vi "BuildExe.vi"(8 "Error In":errorcluster, 9 "Version number":T1, 10 "Build specification name":string, 11 "Path":path) -> (0 "Error Out":errorcluster)   [LabVIEW 2019]
uses:
  <vilib>/AppBuilder/AB_API/common/AB_API Version Number.ctl
  <vilib>/AppBuilder/AB_API/common/AB_API Build Object Selector.ctl
  <vilib>/AppBuilder/AB_API/Build/NI_AB_API_Build.lvclass
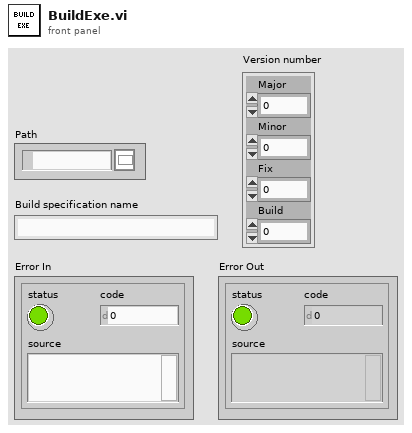
[diagram p1: front panel]
types:
  T1 = typedef "AB_API Version Number.ctl" = cluster{"Major":u16, "Minor":u16, "Fix":u16, "Build":u16}
  T2 = typedef "AB_API Build Object Selector.ctl" = enum16{"Source Distribution", "Deployable Source Distribution", "DLL", "EXE", "Packed Library", "Deployable Packed Library", "RT EXE", ".NET Interop Assembly"}
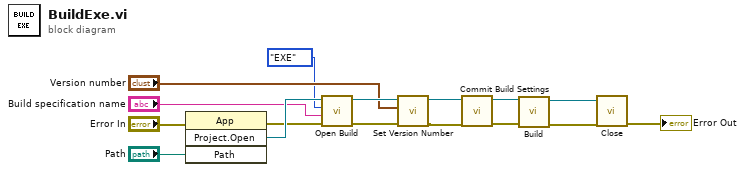
[diagram p0: block diagram]
diagram:
  n1 = invoke class="App" method="Project.Open"(error in="Error In", "Path"="Path") -> (error out=w13:errorcluster, "Project:Open"=w15:refnum<vi>)  [unwired: 2 in, 2 out]
  n2 = call <vilib>:"Open Build.vi"("error in (no error)"=w13, "Build specification name"="Build specification name", "Build object selector"=AB_API_Build_Object_Selector."EXE", "Project Refnum"=w15) -> ("error out"=w9:errorcluster, "NI_AB_API_Build out"=w12:refnum<class "NI_AB_API_Build.lvclass">)  [unwired: 6 in]
  n3 = call-dynamic "Set Version Number.vi"("error in (no error)"=w9, "Version number"="Version number", "NI_AB_API_Targetfile in"=w12) -> ("error out"=w3:errorcluster, "NI_AB_API_Targetfile out"=w4:refnum<class "NI_AB_API_Build.lvclass">)  [unwired: 7 in]
  n4 = call-dynamic "Commit Build Settings.vi"("error in (no error)"=w3, "Build in"=w4) -> ("error out"=w8:errorcluster, "Build out"=w11:refnum<class "NI_AB_API_Build.lvclass">)  [unwired: 8 in]
  n5 = call-dynamic "Build.vi"("error in (no error)"=w8, "Build in"=w11) -> ("error out"=w7:errorcluster, "Build out"=w10:refnum<class "NI_AB_API_Build.lvclass">)  [unwired: 6 in, 2 out]
  n6 = call-dynamic "Close.vi"("error in (no error)"=w7, "NI_AB_API_Build in"=w10) -> ("error out"=→"Error Out":errorcluster)  [unwired: 9 in]
